vi "Lex Set Delimiter Example with More Whitespace.vi"(8 "Error In":errorcluster) -> (0 "Error Out":errorcluster)   [LabVIEW 2018, in "Tests.lvlib" / "Lexer.lvlib"]
uses:
  Lexer.lvlib
  src/Toolkit/Low-Level/Tokens/Text/Text.lvclass
  src/Toolkit/Low-Level/Tokens/EscapedVariable/EscapedVariable.lvclass
  src/Toolkit/Low-Level/Tokens/Keyable/Keyable.lvclass/Keyable.ctl
  src/Toolkit/Low-Level/Tokens/Keyable/Read Key.vi
  src/Toolkit/Low-Level/Support/Lex String.vi
  <vilib>/Utility/LVClass/Get LV Class Name.vi
  src/Toolkit/Low-Level/Tokens/Contentable/Contentable.lvclass
  src/Toolkit/Low-Level/Tokens/Keyable/Keyable.lvclass
  <vilib>/addons/_JKI Toolkits/Caraya/classes/Test/Test.lvclass
  <vilib>/addons/_JKI Toolkits/Caraya/classes/Assert/Assert.lvclass
  Tests.lvlib
  src/Toolkit/Low-Level/Tokens/Abstract/Abstract.lvclass
  src/Toolkit/Toolkit.lvlib
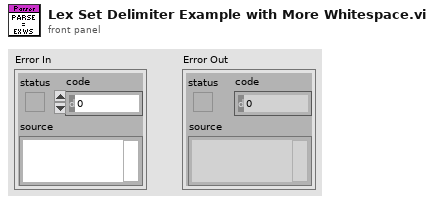
[diagram p1: front panel]
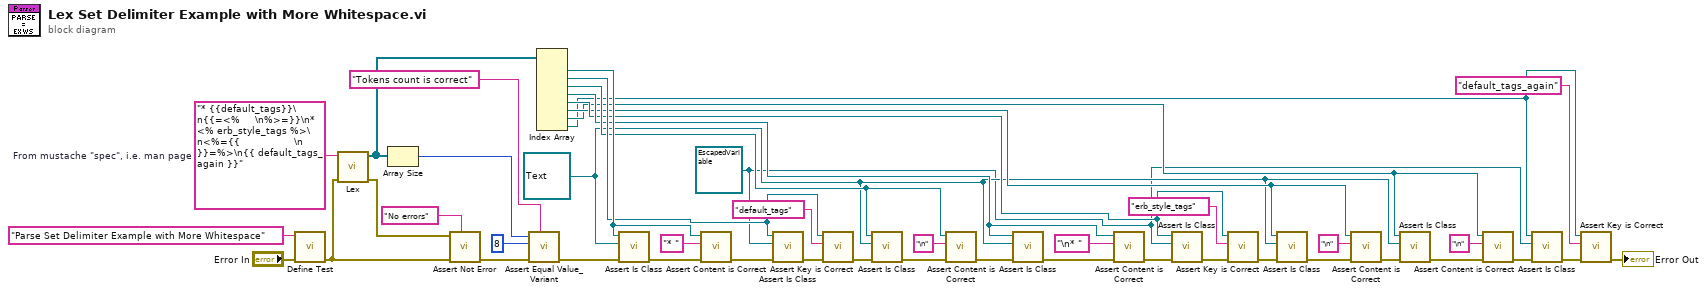
[diagram p0: block diagram]
diagram:
  w5 = refnum<class "EscapedVariable.lvclass"> refnum ("Mustache.lvlib:Tokens.lvlib:EscapedVariable.lvclass")
  w11 = refnum<class "Text.lvclass"> refnum ("Mustache.lvlib:Tokens.lvlib:Text.lvclass")
  w1 = "* {{default_tags}}\n{{=<%     \n%>=}}\n* <% erb_style_tags %>\n<%={{                  \n       }}=%>\n{{ default_tags_again }}"  # From mustache "spec", i.e. man page
  n1 = call <vilib>:"Define Test.vi"("error in (no error)"="Error In", "Label (VI Title)"="Parse Set Delimiter Example with More Whitespace") -> ("error out"=w2:errorcluster)  [unwired: 9 in]
  n2 = call-poly "Lex.vi"("Error In"=w2, "Input"=w1) -> ("Error Out"=w44:errorcluster, "Tokens"=w38:refnum<class "Abstract.lvclass">[])  [unwired: 8 in]
  n3 = Array Size(array=w38) -> (size(s)=w40:i32)
  n4 = call <vilib>:"Assert Not Error.vi"("Label"="No errors", "error in (no error)"=w2, "Not Error?"=w44) -> ("error out"=w42:errorcluster)  [unwired: 8 in]
  n5 = call <vilib>:"Assert Equal Value_Variant.vi"("Label"="Tokens count is correct", "error in (no error)"=w42, "Y"=8 ("size(s)"), "X"=w40) -> ("error out"=w37:errorcluster)  [unwired: 7 in]
  n6 = Index Array(array=w38) -> (element #1=w35:refnum<class "Abstract.lvclass">, element #2=w31:refnum<class "Abstract.lvclass">, element #3=w26:refnum<class "Abstract.lvclass">, element #4=w22:refnum<class "Abstract.lvclass">, element #5=w19:refnum<class "Abstract.lvclass">, element #6=w15:refnum<class "Abstract.lvclass">, element #7=w10:refnum<class "Abstract.lvclass">, element #8=w4:refnum<class "Abstract.lvclass">)  [unwired: 8 in]
  n7 = call "Assert Is Class.vi"("Error In"=w37, "Expected"=w11, "Actual"=w35) -> ("Error Out"=w36:errorcluster)  [unwired: 8 in]
  n8 = call "Assert Content is Correct.vi"("Error In"=w36, "Expected"="* ", "Token"=w35) -> ("Error Out"=w33:errorcluster)  [unwired: 8 in]
  n9 = call "Assert Is Class.vi"("Error In"=w33, "Expected"=w5, "Actual"=w31) -> ("Error Out"=w32:errorcluster)  [unwired: 8 in]
  n10 = call "Assert Key is Correct.vi"("Error In"=w32, "Expected"="default_tags", "Token"=w31) -> ("Error Out"=w29:errorcluster)  [unwired: 8 in]
  n11 = call "Assert Is Class.vi"("Error In"=w29, "Expected"=w11, "Actual"=w26) -> ("Error Out"=w28:errorcluster)  [unwired: 8 in]
  n12 = call "Assert Content is Correct.vi"("Error In"=w28, "Expected"="\n", "Token"=w26) -> ("Error Out"=w25:errorcluster)  [unwired: 8 in]
  n13 = call "Assert Is Class.vi"("Error In"=w25, "Expected"=w11, "Actual"=w22) -> ("Error Out"=w24:errorcluster)  [unwired: 8 in]
  n14 = call "Assert Content is Correct.vi"("Error In"=w24, "Expected"="\n* ", "Token"=w22) -> ("Error Out"=w21:errorcluster)  [unwired: 8 in]
  n15 = call "Assert Is Class.vi"("Error In"=w21, "Expected"=w5, "Actual"=w19) -> ("Error Out"=w20:errorcluster)  [unwired: 8 in]
  n16 = call "Assert Key is Correct.vi"("Error In"=w20, "Expected"="erb_style_tags", "Token"=w19) -> ("Error Out"=w17:errorcluster)  [unwired: 8 in]
  n17 = call "Assert Is Class.vi"("Error In"=w17, "Expected"=w11, "Actual"=w15) -> ("Error Out"=w16:errorcluster)  [unwired: 8 in]
  n18 = call "Assert Content is Correct.vi"("Error In"=w16, "Expected"="\n", "Token"=w15) -> ("Error Out"=w13:errorcluster)  [unwired: 8 in]
  n19 = call "Assert Is Class.vi"("Error In"=w13, "Expected"=w11, "Actual"=w10) -> ("Error Out"=w12:errorcluster)  [unwired: 8 in]
  n20 = call "Assert Content is Correct.vi"("Error In"=w12, "Expected"="\n", "Token"=w10) -> ("Error Out"=w8:errorcluster)  [unwired: 8 in]
  n21 = call "Assert Is Class.vi"("Error In"=w8, "Expected"=w5, "Actual"=w4) -> ("Error Out"=w7:errorcluster)  [unwired: 8 in]
  n22 = call "Assert Key is Correct.vi"("Error In"=w7, "Expected"="default_tags_again", "Token"=w4) -> ("Error Out"=→"Error Out":errorcluster)  [unwired: 8 in]
